vi "ProtoGenerator.vi"(8 "error in (no error)":errorcluster, 11 ".proto file path":path=path "C:/dev/labview-grpc-server/tests/data_marshal/data_marshal.proto") -> (0 "error out":errorcluster, 1 "gRPC Method Parameters":T4[](array[typedef]), 2 "gRPC Messages Parameters":T1[](array[typedef]))   [LabVIEW 2019, in "gRPC Scripting Tools.lvlib"]
uses:
  gRPC Scripting Tools.lvlib
  TypeDefs/RPC Method Parameters.ctl
  TypeDefs/Message Metadata (Scripting).ctl
  TypeDefs/Message Element Metadata (Scripting).ctl
  TypeDefs/Message Element Type.ctl
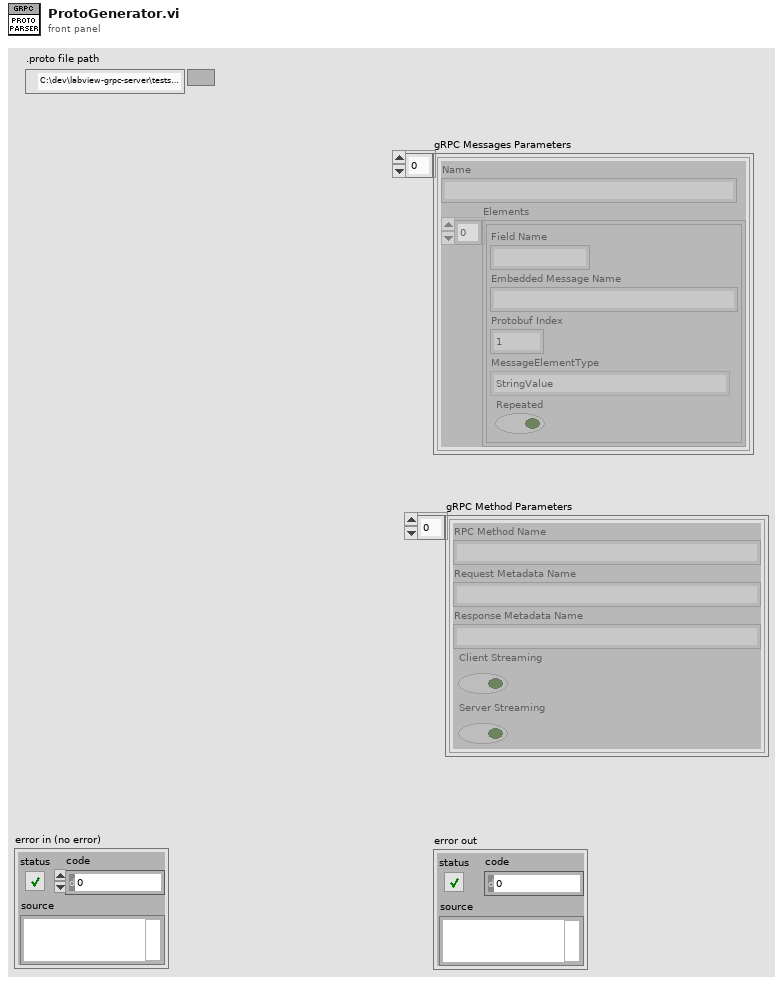
[diagram p1: front panel]
types:
  T1 = typedef "gRPC Scripting Tools.lvlib/Message Metadata (Scripting).ctl" = cluster{"Name":string, "Elements":T2[]}
  T2 = typedef "gRPC Scripting Tools.lvlib/Message Element Metadata (Scripting).ctl" = cluster{"Field Name":string, "Embedded Message Name":string, "Protobuf Index":i32, "MessageElementType":T3, "Repeated":bool}
  T3 = typedef "gRPC Scripting Tools.lvlib/Message Element Type.ctl" = enum32{"Int32Value", "FloatValue", "DoubleValue", "BoolValue", "StringValue", "MessageValue", ""}
  T4 = typedef "gRPC Scripting Tools.lvlib/RPC Method Parameters.ctl" = cluster{"RPC Method Name":string, "Request Metadata Name":string, "Response Metadata Name":string, "Client Streaming":bool, "Server Streaming":bool}
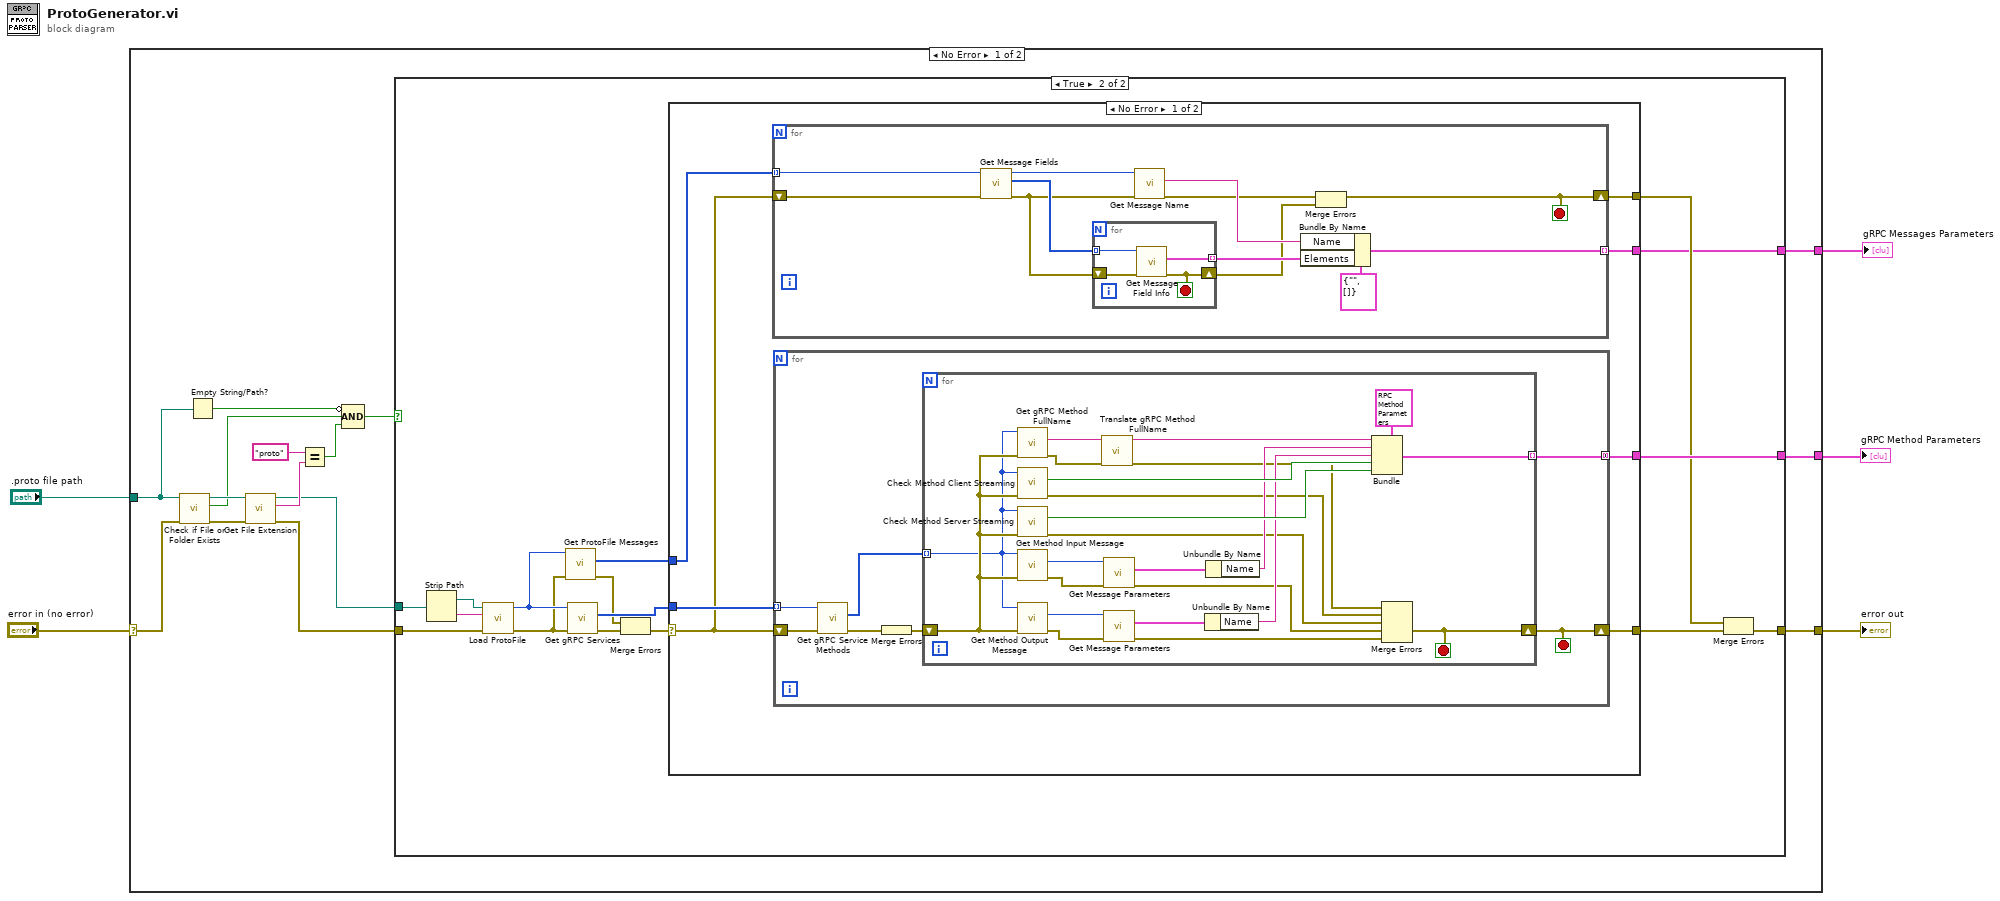
[diagram p0: block diagram]
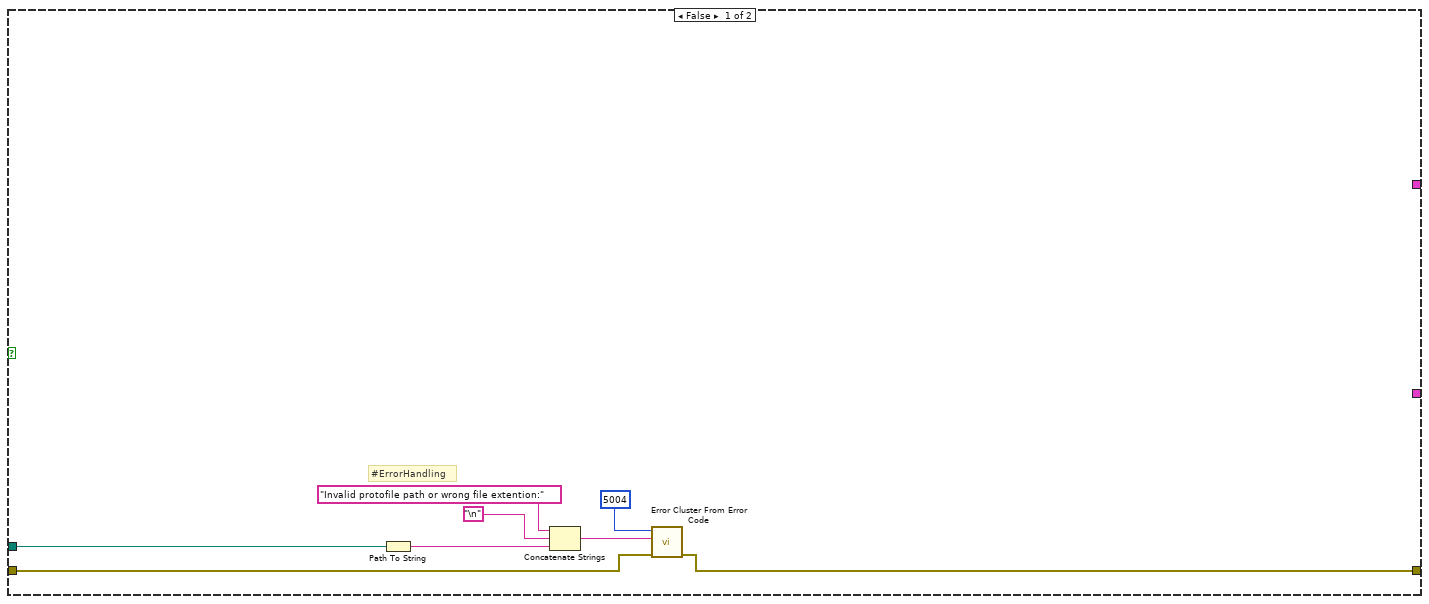
[diagram p2: hidden frame]
diagram:
  n1 = case shown="No Error" "error in (no error)" {
    selector: "error in (no error)" -> [w17 w99]
    tunnel: ".proto file path" -> [w18 _]
    tunnel: [w20 _] -> w5
    tunnel: [w19 w99] -> w4
    tunnel: [w6 _] -> w1
    frame No Error {
      n2 = call <vilib>:"Check if File or Folder Exists.vi"("error in (no error)"=w17, "path"=w18) -> ("error out"=w16:errorcluster, "file or folder exists?"=w11:bool, "dup path"=w15:path)  [unwired: 7 in]
      n3 = Empty String/Path?(string/path=w18) -> (empty?=w10:bool)
      n4 = call <vilib>:"Get File Extension.vi"("error in (no error)"=w16, "file"=w15) -> ("error out"=w7:errorcluster, "lowercase file extension"=w14:string, "dup file"=w8:path)  [unwired: 5 in, 2 out]
      n5 = Equal?(x="proto", y=w14) -> (x = y?=w12:bool)
      n6 = Compound Arithmetic op=AND(invert w10, w11, w12) -> (w9:bool)
      n7 = case shown="True" w9 {
        tunnel: [_ w41] -> w20
        tunnel: [w21 w30] -> w19
        tunnel: w8 -> [w24 w40]
        tunnel: w7 -> [w27 w39]
        tunnel: [_ w29] -> w6
        frame False {
          # "#ErrorHandling"
          n8 = Path To String(path=w24) -> (string=w23:string)
          n9 = Concatenate Strings("Invalid protofile path or wrong file extention:" ("error message (\"\")"), "\n", w23) -> (w22:string)
          n10 = call <vilib>:"Error Cluster From Error Code.vi"("error in (no error)"=w27, "error message (\"\")"=w22, "error code (0)"=5004) -> ("error out"=w21:errorcluster)  [unwired: 6 in]
        }
        frame True {
          n11 = Strip Path(path=w40) -> (stripped path=w44:path, name=w43:string)
          n12 = call "Load ProtoFile.vi"("error in (no error)"=w39, "File Name"=w43, "File Base path"=w44) -> ("error out"=w36:errorcluster, "protoFile ref out"=w37:u64)  [unwired: 7 in]
          n13 = call "Get ProtoFile Messages.vi"("error in (no error)"=w36, "Protofile ref in"=w37) -> ("error out"=w35:errorcluster, "ProtoFile Messages"=w33:u64[])  [unwired: 7 in, 1 out]
          n14 = call "Get gRPC Services.vi"("error in (no error)"=w36, "protoFile ref in"=w37) -> ("error out"=w38:errorcluster, "services"=w42:u64[])  [unwired: 7 in, 1 out]
          n15 = Merge Errors(w35, w38) -> (w34:errorcluster)
          n16 = case shown="No Error" w34 {
            selector: w34 -> [w47 w98]
            tunnel: w42 -> [w51 _]
            tunnel: [w50 _] -> w41
            tunnel: [w49 w98] -> w32
            tunnel: w33 -> [w48 _]
            tunnel: [w46 _] -> w31
            tunnel: [w45 _] -> w29
            frame No Error {
              n17 = for {
                tunnel: w48 -> [w63] mode=indexing
                shift-right: [w52] -> w46
                shift-left: w47 -> [w57]
                tunnel: [w53] -> w45 mode=indexing
                stop <- w52 stop-if-true
                n18 = call "Get Message Fields.vi"("error in (no error)"=w57, "Message ref in"=w63) -> ("error out"=w56:errorcluster, "Field refs"=w62:u64[], "Message ref out"=w61:u64)  [unwired: 7 in]
                n19 = for {
                  tunnel: w62 -> [w67] mode=indexing
                  tunnel: [w66] -> w58 mode=indexing
                  shift-right: [w64] -> w55
                  shift-left: w56 -> [w65]
                  stop <- w64 stop-if-true
                  n20 = call "Get Message Field Info.vi"("error in (no error)"=w65, "Message Field ref in"=w67) -> ("error out"=w64:errorcluster, "Field Info"=w66:T2)  [unwired: 7 in, 1 out]
                }
                n21 = call "Get Message Name.vi"("error in (no error)"=w56, "Message ref in"=w61) -> ("error out"=w54:errorcluster, "Message Name"=w59:string)  [unwired: 7 in, 1 out]
                n22 = Bundle By Name(cluster=T1 {"Name"="", "Elements"=[]} ("Message Metadata"), "Name"=w59, "Elements"=w58) -> (w53:T1)
                n23 = Merge Errors(w54, w55) -> (w52:errorcluster)
              }
              n24 = for {
                tunnel: w51 -> [w74] mode=indexing
                tunnel: [w73] -> w50 mode=concatenating
                shift-right: [w68] -> w49
                shift-left: w47 -> [w71]
                stop <- w68 stop-if-true
                n25 = call "Get gRPC Service Methods.vi"("error in (no error)"=w71, "Service ref in"=w74) -> ("error out"=w70:errorcluster, "Service Methods"=w72:u64[])  [unwired: 7 in, 1 out]
                n26 = Merge Errors(w70) -> (w69:errorcluster)
                n27 = for {
                  tunnel: w72 -> [w79] mode=indexing
                  tunnel: [w97] -> w73 mode=indexing
                  shift-right: [w81] -> w68
                  shift-left: w69 -> [w80]
                  stop <- w81 stop-if-true
                  n28 = call "Get gRPC Method FullName.vi"("error in (no error)"=w80, "Method ref in"=w79) -> ("error out"=w78:errorcluster, "Method Full Name"=w77:string)  [unwired: 7 in, 1 out]
                  n29 = call "Check Method Client Streaming.vi"("error in (no error)"=w80, "Method ref in"=w79) -> ("error out"=w85:errorcluster, "is Client Streaming"=w96:bool)  [unwired: 7 in, 1 out]
                  n30 = call "Check Method Server Streaming.vi"("error in (no error)"=w80, "Method ref in"=w79) -> ("error out"=w84:errorcluster, "is Server Streaming"=w95:bool)  [unwired: 7 in, 1 out]
                  n31 = call "Get Method Input Message.vi"("error in (no error)"=w80, "Method ref in"=w79) -> ("error out"=w90:errorcluster, "Message ref out"=w93:u64)  [unwired: 7 in, 1 out]
                  n32 = call "Get Method Output Message.vi"("error in (no error)"=w80, "Method ref in"=w79) -> ("error out"=w91:errorcluster, "Message ref out"=w92:u64)  [unwired: 7 in, 1 out]
                  n33 = call "Translate gRPC Method FullName.vi"("error in (no error)"=w78, "Method Full Name in"=w77) -> ("error out"=w75:errorcluster, "Method Full Name out"=w76:string)  [unwired: 8 in]
                  n34 = call "Get Message Parameters.vi"("error in (no error)"=w90, "Message ref in"=w93) -> ("error out"=w83:errorcluster, "Message Metadata"=w87:T1)  [unwired: 7 in, 1 out]
                  n35 = call "Get Message Parameters.vi"("error in (no error)"=w91, "Message ref in"=w92) -> ("error out"=w82:errorcluster, "Message Metadata"=w86:T1)  [unwired: 7 in, 1 out]
                  n36 = Unbundle By Name(w86) -> ("Name"=w88:string)
                  n37 = Unbundle By Name(w87) -> ("Name"=w89:string)
                  n38 = Bundle(cluster=T4 {"RPC Method Name"="/queryserver.QueryServer/Invoke", "Request Metadata Name"="InvokeRequest", "Response Metadata Name"="InvokeResponse", "Client Streaming"=FALSE, "Server Streaming"=FALSE}, "RPC Method Name"=w76, "Request Metadata Name"=w89, "Response Metadata Name"=w88, "Client Streaming"=w96, "Server Streaming"=w95) -> (w97:T4)
                  n39 = Merge Errors(w75, w85, w84, w83, w82) -> (w81:errorcluster)
                }
              }
            }
            frame Error {
            }
          }
          n40 = Merge Errors(w31, w32) -> (w30:errorcluster)
        }
      }
    }
    frame Error {
    }
  }
  "gRPC Method Parameters" <- w5
  "error out" <- w4
  "gRPC Messages Parameters" <- w1
